vi "Byte_to_DeviceConfigType.vi"(4 "Byte Array":u8[](array[numeric])) -> (1 "output cluster":T1)   [LabVIEW 2020]
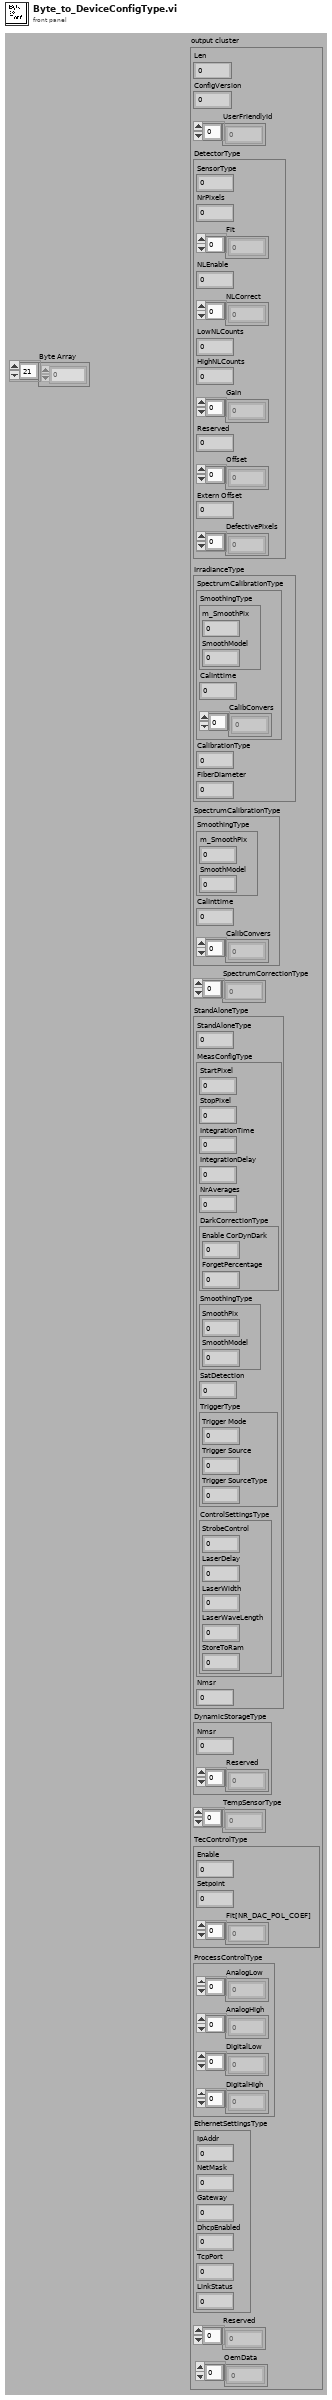
[diagram p1: front panel]
types:
  T1 = cluster{"Len":u16, "ConfigVersion":u16, "UserFriendlyId":u8[], "DetectorType":cluster{"SensorType":u8, "NrPixels":u16, "Fit":sgl[], "NLEnable":u8, "NLCorrect":dbl[], "LowNLCounts":dbl, "HighNLCounts":dbl, "Gain":sgl[], "Reserved":sgl, "Offset":sgl[], "Extern Offset":sgl, "DefectivePixels":u16[]}, "IrradianceType":cluster{"SpectrumCalibrationType":cluster{"SmoothingType":cluster{"m_SmoothPix":u16, "SmoothModel":u8}, "CalInttime":sgl, "CalibConvers":sgl[]}, "CalibrationType":u8, "FiberDiameter":i32}, "SpectrumCalibrationType":cluster{"SmoothingType":cluster{"m_SmoothPix":u16, "SmoothModel":u8}, "CalInttime":sgl, "CalibConvers":sgl[]}, "SpectrumCorrectionType":sgl[], "StandAloneType":cluster{"StandAloneType":u8, "MeasConfigType":cluster{"StartPixel":u16, "StopPixel":u16, "IntegrationTime":sgl, "IntegrationDelay":u32, "NrAverages":u32, "DarkCorrectionType":cluster{"Enable CorDynDark":u8, "ForgetPercentage":u8}, "SmoothingType":cluster{"SmoothPix":u16, "SmoothModel":u8}, "SatDetection":u8, "TriggerType":cluster{"Trigger Mode":u8, "Trigger Source":u8, "Trigger SourceType":u8}, "ControlSettingsType":cluster{"StrobeControl":u16, "LaserDelay":u32, "LaserWidth":u32, "LaserWaveLength":sgl, "StoreToRam":u16}}, "Nmsr":i16}, "DynamicStorageType":cluster{"Nmsr":i32, "Reserved":u8[]}, "TempSensorType":sgl[], "TecControlType":cluster{"Enable":u8, "Setpoint":sgl, "Fit[NR_DAC_POL_COEF]":sgl[]}, "ProcessControlType":cluster{"AnalogLow":sgl[], "AnalogHigh":sgl[], "DigitalLow":sgl[], "DigitalHigh":sgl[]}, "EthernetSettingsType":cluster{"IpAddr":u32, "NetMask":u32, "Gateway":u32, "DhcpEnabled":u8, "TcpPort":u16, "LinkStatus":u8}, "Reserved":u8[], "OemData":u8[]}
  T2 = cluster{"Len":u16, "ConfigVersion":u16, "UserFriendlyId":u8[], "DetectorType":cluster{"SensorType":u8, "NrPixels":u16, "Fit":sgl[], "NLEnable":u8, "NLCorrect":dbl[], "LowNLCounts":dbl, "HighNLCounts":dbl, "Gain":sgl[], "Reserved":sgl, "Offset":sgl[], "Extern Offset":sgl, "DefectivePixels":u16[]}, "IrradianceType":cluster{"SpectrumCalibrationType":cluster{"SmoothingType":cluster{"m_SmoothPix":u16, "SmoothModel":u8}, "CalInttime":sgl, "CalibConvers":sgl[]}, "CalibrationType":u8, "FiberDiameter":i32}, "SpectrumCalibrationType":cluster{"SmoothingType":cluster{"m_SmoothPix":u16, "SmoothModel":u8}, "CalInttime":sgl, "CalibConvers":sgl[]}, "SpectrumCorrectionType":sgl[], "StandAloneType":cluster{"StandAloneType":u8, "MeasConfigType":cluster{"StartPixel":u16, "StopPixel":u16, "IntegrationTime":sgl, "IntegrationDelay":u32, "NrAverages":u32, "DarkCorrectionType":cluster{"Enable CorDynDark":u8, "ForgetPercentage":u8}, "SmoothingType":cluster{"SmoothPix":u16, "SmoothModel":u8}, "SatDetection":u8, "TriggerType":cluster{"Trigger Mode":u8, "Trigger Source":u8, "Trigger SourceType":u8}, "ControlSettingsType":cluster{"StrobeControl":u16, "LaserDelay":u32, "LaserWidth":u32, "LaserWaveLength":sgl, "StoreToRam":u16}}, "Nmsr":i16}, "DynamicStorageType":cluster{"Nmsr":i32, "Reserved":u8[]}, "TempSensorType":sgl[], "TecControlType":cluster{"Enable":u8, "Setpoint":sgl, "Fit[NR_DAC_POL_COEF]":sgl[]}, "ProcessControlType\n":cluster{"AnalogLow":sgl[], "AnalogHigh":sgl[], "DigitalLow":sgl[], "DigitalHigh":sgl[]}, "EthernetSettingsType":cluster{"IpAddr":u32, "NetMask":u32, "Gateway":u32, "DhcpEnabled":u8, "TcpPort":u16, "LinkStatus":u8}, "Reserved":u8[], "OemData":u8[]}
  T3 = cluster{u8, u16, sgl[], u8, dbl[], dbl, dbl, sgl[], sgl, sgl[], sgl, u16[]}
  T4 = cluster{cluster{cluster{u16, u8}, sgl, sgl[]}, u8, i32}
  T5 = cluster{u16, u16, sgl, u32, u32, cluster{u8, u8}, cluster{u16, u8}, u8, cluster{u8, u8, u8}, cluster{u16, u32, u32, sgl, u16}}
  T6 = cluster{u8, cluster{u16, u16, sgl, u32, u32, cluster{u8, u8}, cluster{u16, u8}, u8, cluster{u8, u8, u8}, cluster{u16, u32, u32, sgl, u16}}, i16}
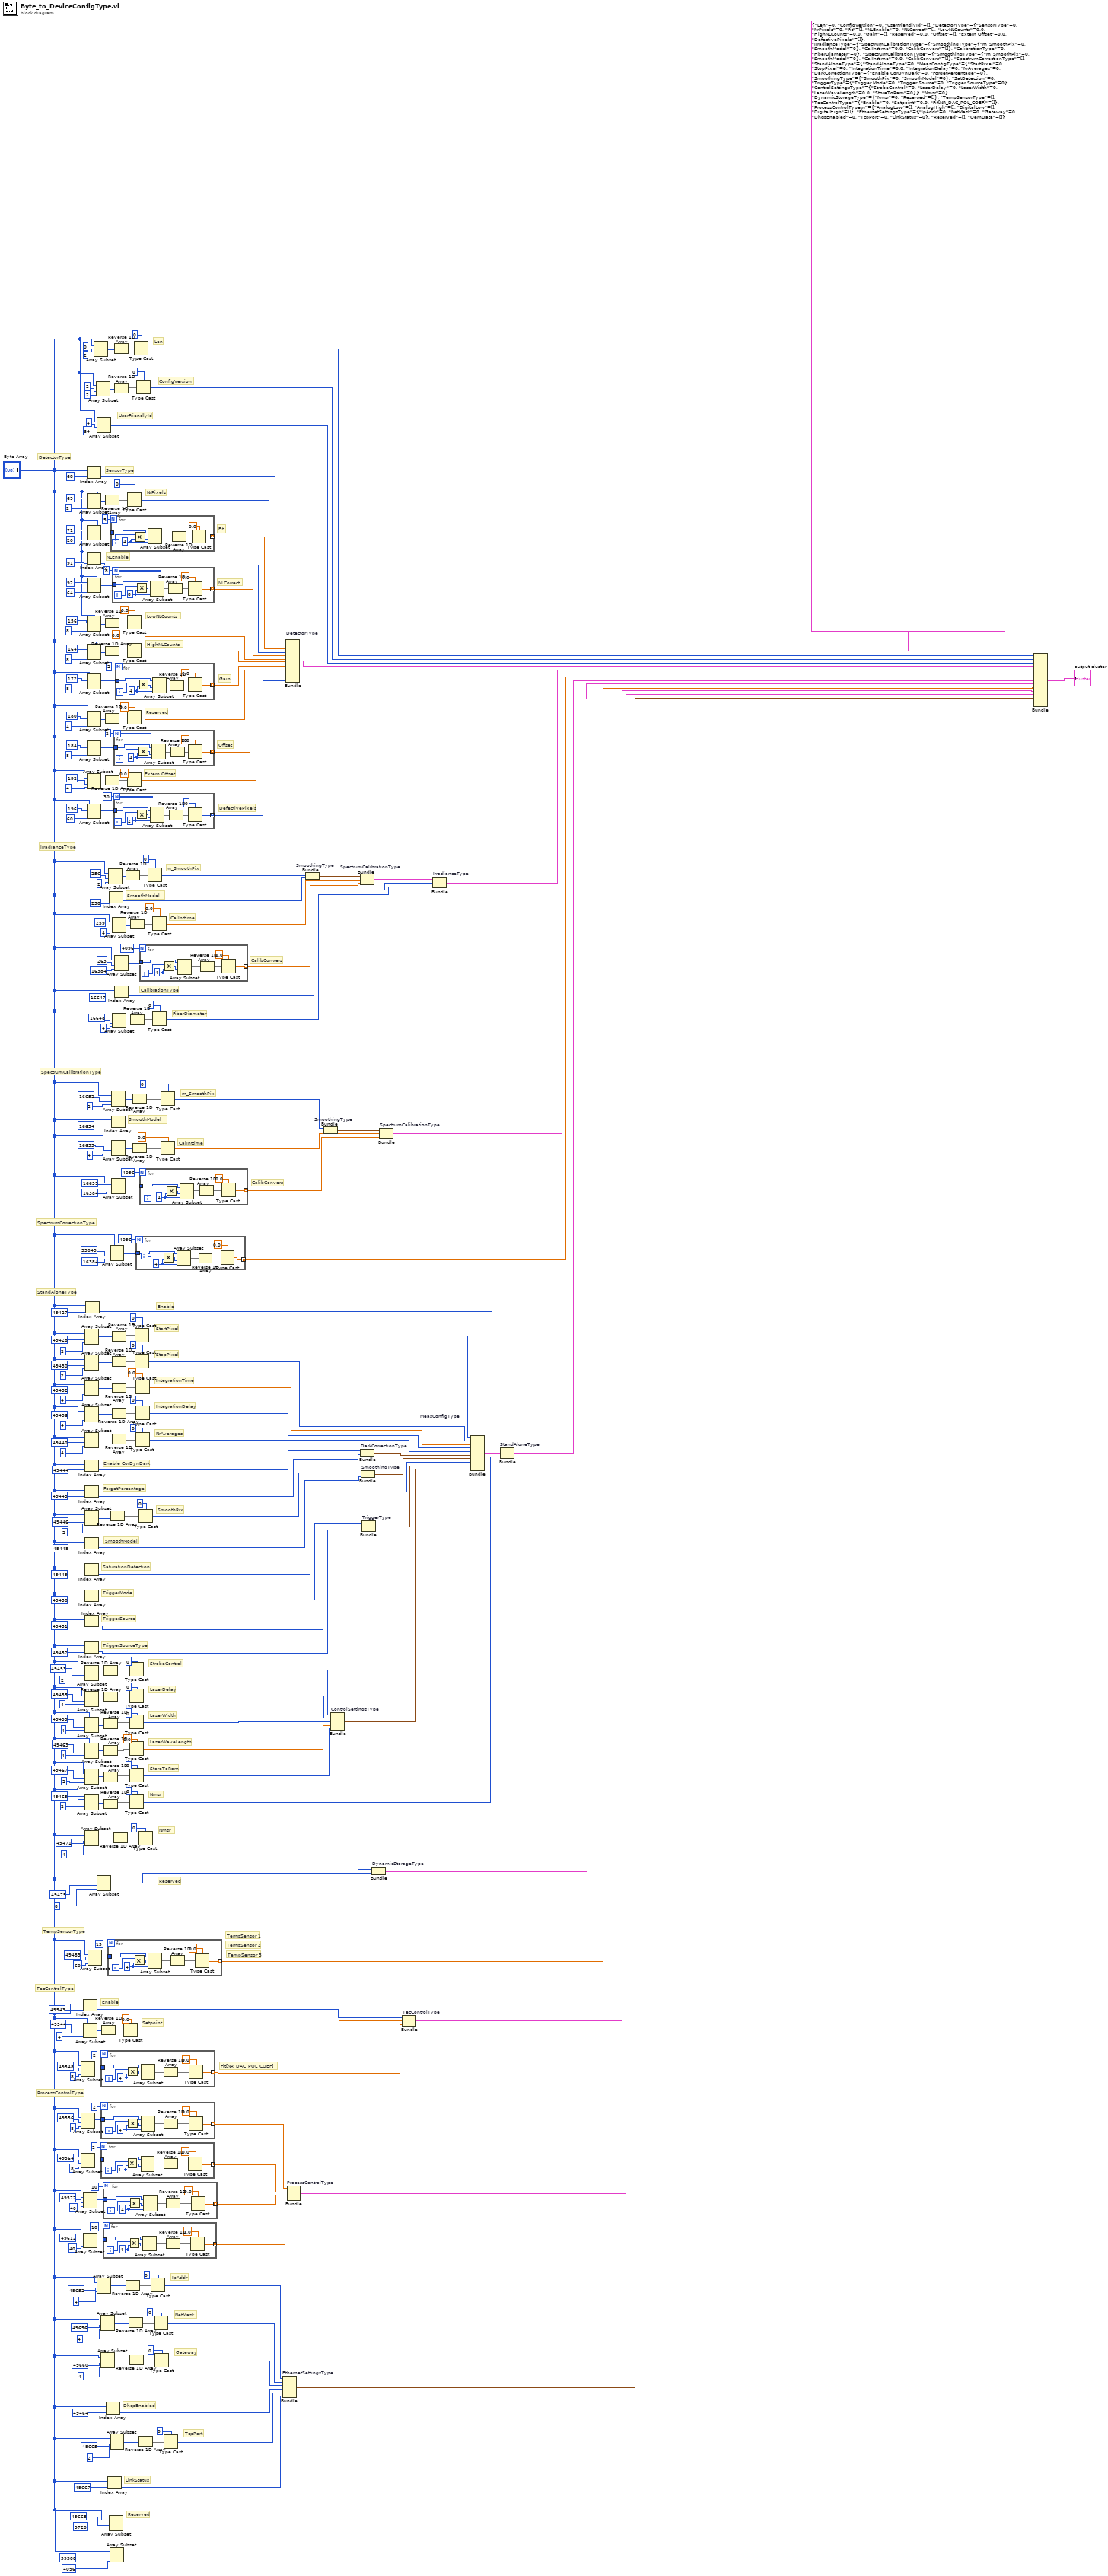
[diagram p0: block diagram]
diagram:
  # "Enable"
  # "LinkStatus"
  # "DhcpEnabled"
  # "TcpPort"
  # "Gateway"
  # "NetMask"
  # "IpAddr"
  # "ProcessControlType"
  # "TecControlType"
  # "Len"
  # "ConfigVersion"
  # "Fit[NR_DAC_POL_COEF]"
  # "Setpoint"
  # "Enable"
  # "UserFriendlyId"
  # "SensorType"
  # "NrPixels"
  # "Fit"
  # "NLEnable"
  # "NLCorrect"
  # "LowNLCounts"
  # "HighNLCounts"
  # "Gain"
  # "Offset"
  # "DetectorType"
  # "TempSensor 3"
  # "TempSensor 2"
  # "Reserved"
  # "TempSensor 1"
  # "TempSensorType"
  # "Reserved"
  # "Nmsr"
  # "Nmsr"
  # "StoreToRam"
  # "LaserWaveLength"
  # "LaserWidth"
  # "LaserDelay"
  # "StrobeControl"
  # "TriggerSourceType"
  # "TriggerSource"
  # "TriggerMode"
  # "SaturationDetection"
  # "SmoothModel"
  # "SmoothPix"
  # "ForgetPercentage"
  # "Enable CorDynDark"
  # "NrAverages"
  # "IntegrationDelay"
  # "IntegrationTime"
  # "StopPixel"
  # "StartPixel"
  # "StandAloneType"
  # "SpectrumCorrectionType"
  # "CalibConvers"
  # "CalInttime"
  # "SmoothModel"
  # "m_SmoothPix"
  # "SpectrumCalibrationType"
  # "FiberDiameter"
  # "CalibrationType"
  # "CalibConvers"
  # "CalInttime"
  # "SmoothModel"
  # "IrradianceType"
  # "m_SmoothPix"
  # "DefectivePixels"
  # "Reserved"
  # "Extern Offset"
  n1 = Array Subset(array="Byte Array", index=49564, length=8) -> (w62:u8[])
  n2 = Array Subset(array="Byte Array", index=49548, length=8) -> (w71:u8[])
  n3 = Array Subset(array="Byte Array", index=49556, length=8) -> (w66:u8[])
  n4 = Index Array(array="Byte Array", index=49543 ("length")) -> (element=w78:u8)
  n5 = Array Subset(array="Byte Array", index=49612, length=40) -> (w54:u8[])
  n6 = Array Subset(array="Byte Array", index=49544, length=4) -> (w74:u8[])
  n7 = Array Subset(array="Byte Array", index=49572, length=40) -> (w58:u8[])
  n8 = Array Subset(array="Byte Array", index=49471 ("length"), length=4) -> (w45:u8[])
  n9 = Array Subset(array="Byte Array", index=49428, length=2) -> (w222:u8[])
  n10 = Array Subset(array="Byte Array", index=49430, length=2) -> (w217:u8[])
  n11 = Array Subset(array="Byte Array", index=49432, length=4) -> (w214:u8[])
  n12 = Array Subset(array="Byte Array", index=49436, length=4) -> (w205:u8[])
  n13 = Array Subset(array="Byte Array", index=49440, length=4) -> (w202:u8[])
  n14 = Index Array(array="Byte Array", index=49444 ("length")) -> (element=w97:u8)
  n15 = Index Array(array="Byte Array", index=49445 ("length")) -> (element=w96:u8)
  n16 = Array Subset(array="Byte Array", index=49446, length=2) -> (w196:u8[])
  n17 = Index Array(array="Byte Array", index=49448 ("length")) -> (element=w94:u8)
  n18 = Index Array(array="Byte Array", index=49449 ("length")) -> (element=w93:u8)
  n19 = Index Array(array="Byte Array", index=49450 ("length")) -> (element=w92:u8)
  n20 = Index Array(array="Byte Array", index=49451 ("length")) -> (element=w91:u8)
  n21 = Index Array(array="Byte Array", index=49452 ("length")) -> (element=w90:u8)
  n22 = Array Subset(array="Byte Array", index=49453, length=2) -> (w184:u8[])
  n23 = Array Subset(array="Byte Array", index=49455, length=4) -> (w181:u8[])
  n24 = Array Subset(array="Byte Array", index=49459, length=4) -> (w174:u8[])
  n25 = Array Subset(array="Byte Array", index=49463, length=4) -> (w171:u8[])
  n26 = Array Subset(array="Byte Array", index=49467, length=2) -> (w164:u8[])
  n27 = Array Subset(array="Byte Array", index=49469, length=2) -> (w159:u8[])
  n28 = Index Array(array="Byte Array", index=49427 ("length")) -> (element=w103:u8)
  n29 = Index Array(array="Byte Array", index=68 ("length")) -> (element=w136:u8)
  n30 = Array Subset(array="Byte Array", index=69, length=2) -> (w300:u8[])
  n31 = Array Subset(array="Byte Array", index=71, length=20) -> (w133:u8[])
  n32 = Index Array(array="Byte Array", index=91 ("length")) -> (element=w132:u8)
  n33 = Array Subset(array="Byte Array", index=92, length=64) -> (w130:u8[])
  n34 = Array Subset(array="Byte Array", index=156, length=8) -> (w286:u8[])
  n35 = Array Subset(array="Byte Array", index=164, length=8) -> (w283:u8[])
  n36 = Array Subset(array="Byte Array", index=172, length=8) -> (w126:u8[])
  n37 = Array Subset(array="Byte Array", index=180, length=4) -> (w274:u8[])
  n38 = Array Subset(array="Byte Array", index=184, length=8) -> (w123:u8[])
  n39 = Array Subset(array="Byte Array", index=192, length=4) -> (w266:u8[])
  n40 = Array Subset(array="Byte Array", index=196, length=60) -> (w121:u8[])
  n41 = Array Subset(array="Byte Array", index=49483, length=60) -> (w81:u8[])
  n42 = Array Subset(array="Byte Array", index=0, length=2) -> (w305:u8[])
  n43 = Array Subset(array="Byte Array", index=2, length=2) -> (w304:u8[])
  n44 = Array Subset(array="Byte Array", index=4, length=64) -> (w137:u8[])
  n45 = Array Subset(array="Byte Array", index=49475, length=8) -> (w80:u8[])
  n46 = Array Subset(array="Byte Array", index=49652 ("length"), length=4) -> (w38:u8[])
  n47 = for {
    N: 2 -> [_]
    tunnel: w62 -> [w318]
    tunnel: [w316] -> w49 mode=indexing
    i -> [w319]
    w320 = 4 ("length")
    n48 = Multiply(x=w319, y=w320) -> (x*y=w321:i32)
    n49 = Array Subset(array=w318, index=w321, length=w320) -> (w314:u8[])
    n50 = Reverse 1D Array(array=w314) -> (reversed array=w315:u8[])
    n51 = Type Cast(type=sgl 0.0, x=w315) -> (*(type *) &x=w316:sgl)
  }
  n52 = Array Subset(array="Byte Array", index=49656 ("length"), length=4) -> (w33:u8[])
  n53 = for {
    N: 2 -> [_]
    tunnel: w71 -> [w326]
    tunnel: [w324] -> w67 mode=indexing
    i -> [w327]
    w328 = 4 ("length")
    n54 = Multiply(x=w327, y=w328) -> (x*y=w329:i32)
    n55 = Array Subset(array=w326, index=w329, length=w328) -> (w322:u8[])
    n56 = Reverse 1D Array(array=w322) -> (reversed array=w323:u8[])
    n57 = Type Cast(type=sgl 0.0, x=w323) -> (*(type *) &x=w324:sgl)
  }
  n58 = for {
    N: 2 -> [_]
    tunnel: w66 -> [w334]
    tunnel: [w332] -> w50 mode=indexing
    i -> [w335]
    w336 = 4 ("length")
    n59 = Multiply(x=w335, y=w336) -> (x*y=w337:i32)
    n60 = Array Subset(array=w334, index=w337, length=w336) -> (w330:u8[])
    n61 = Reverse 1D Array(array=w330) -> (reversed array=w331:u8[])
    n62 = Type Cast(type=sgl 0.0, x=w331) -> (*(type *) &x=w332:sgl)
  }
  n63 = Array Subset(array="Byte Array", index=49660 ("length"), length=4) -> (w28:u8[])
  n64 = Reverse 1D Array(array=w74) -> (reversed array=w73:u8[])
  n65 = for {
    N: 10 -> [_]
    tunnel: w54 -> [w342]
    tunnel: [w340] -> w47 mode=indexing
    i -> [w343]
    w344 = 4 ("length")
    n66 = Multiply(x=w343, y=w344) -> (x*y=w345:i32)
    n67 = Array Subset(array=w342, index=w345, length=w344) -> (w338:u8[])
    n68 = Reverse 1D Array(array=w338) -> (reversed array=w339:u8[])
    n69 = Type Cast(type=sgl 0.0, x=w339) -> (*(type *) &x=w340:sgl)
  }
  n70 = for {
    N: 10 -> [_]
    tunnel: w58 -> [w350]
    tunnel: [w348] -> w48 mode=indexing
    i -> [w351]
    w352 = 4 ("length")
    n71 = Multiply(x=w351, y=w352) -> (x*y=w353:i32)
    n72 = Array Subset(array=w350, index=w353, length=w352) -> (w346:u8[])
    n73 = Reverse 1D Array(array=w346) -> (reversed array=w347:u8[])
    n74 = Type Cast(type=sgl 0.0, x=w347) -> (*(type *) &x=w348:sgl)
  }
  n75 = Reverse 1D Array(array=w184) -> (reversed array=w183:u8[])
  n76 = Reverse 1D Array(array=w181) -> (reversed array=w182:u8[])
  n77 = Reverse 1D Array(array=w174) -> (reversed array=w173:u8[])
  n78 = Reverse 1D Array(array=w171) -> (reversed array=w172:u8[])
  n79 = Reverse 1D Array(array=w164) -> (reversed array=w165:u8[])
  n80 = Reverse 1D Array(array=w159) -> (reversed array=w158:u8[])
  n81 = Reverse 1D Array(array=w300) -> (reversed array=w301:u8[])
  n82 = Reverse 1D Array(array=w286) -> (reversed array=w285:u8[])
  n83 = Reverse 1D Array(array=w283) -> (reversed array=w284:u8[])
  n84 = Reverse 1D Array(array=w274) -> (reversed array=w273:u8[])
  n85 = Reverse 1D Array(array=w266) -> (reversed array=w267:u8[])
  n86 = Index Array(array="Byte Array", index=49464 ("length")) -> (element=w14:u8)
  n87 = for {
    N: 15 -> [_]
    tunnel: w81 -> [w358]
    tunnel: [w356] -> w7 mode=indexing
    i -> [w359]
    w360 = 4 ("length")
    n88 = Multiply(x=w359, y=w360) -> (x*y=w361:i32)
    n89 = Array Subset(array=w358, index=w361, length=w360) -> (w354:u8[])
    n90 = Reverse 1D Array(array=w354) -> (reversed array=w355:u8[])
    n91 = Type Cast(type=sgl 0.0, x=w355) -> (*(type *) &x=w356:sgl)
  }
  n92 = Index Array(array="Byte Array", index=49667 ("length")) -> (element=w12:u8)
  n93 = Array Subset(array="Byte Array", index=256, length=2) -> (w257:u8[])
  n94 = Index Array(array="Byte Array", index=258 ("length")) -> (element=w118:u8)
  n95 = Array Subset(array="Byte Array", index=49668, length=9720) -> (w11:u8[])
  n96 = Array Subset(array="Byte Array", index=59388, length=4096) -> (w3:u8[])
  n97 = for {
    N: 5 -> [_]
    tunnel: w133 -> [w366]
    tunnel: [w364] -> w134 mode=indexing
    i -> [w367]
    w368 = 4 ("length")
    n98 = Multiply(x=w367, y=w368) -> (x*y=w369:i32)
    n99 = Array Subset(array=w366, index=w369, length=w368) -> (w363:u8[])
    n100 = Reverse 1D Array(array=w363) -> (reversed array=w362:u8[])
    n101 = Type Cast(type=sgl 0.0, x=w362) -> (*(type *) &x=w364:sgl)
  }
  n102 = Array Subset(array="Byte Array", index=33043, length=16384) -> (w89:u8[])
  n103 = Array Subset "Array Subset"(array="Byte Array", index=49665 ("length"), length=2) -> (w20:u8[])
  n104 = Reverse 1D Array(array=w196) -> (reversed array=w197:u8[])
  n105 = Array Subset(array="Byte Array", index=16652, length=2) -> (w231:u8[])
  n106 = Index Array(array="Byte Array", index=16654 ("length")) -> (element=w110:u8)
  n107 = Array Subset(array="Byte Array", index=16655, length=4) -> (w234:u8[])
  n108 = Array Subset(array="Byte Array", index=16659, length=16384) -> (w88:u8[])
  n109 = Reverse 1D Array(array=w222) -> (reversed array=w223:u8[])
  n110 = Reverse 1D Array(array=w217) -> (reversed array=w216:u8[])
  n111 = Reverse 1D Array(array=w214) -> (reversed array=w215:u8[])
  n112 = Reverse 1D Array(array=w205) -> (reversed array=w204:u8[])
  n113 = Reverse 1D Array(array=w202) -> (reversed array=w203:u8[])
  n114 = for {
    N: 8 -> [_]
    tunnel: w130 -> [w374]
    tunnel: [w372] -> w131 mode=indexing
    i -> [w375]
    w376 = 8 ("length")
    n115 = Multiply(x=w375, y=w376) -> (x*y=w377:i32)
    n116 = Array Subset(array=w374, index=w377, length=w376) -> (w371:u8[])
    n117 = Reverse 1D Array(array=w371) -> (reversed array=w370:u8[])
    n118 = Type Cast(type=0.0, x=w370) -> (*(type *) &x=w372:dbl)
  }
  n119 = Array Subset(array="Byte Array", index=259, length=4) -> (w253:u8[])
  n120 = Array Subset(array="Byte Array", index=16648, length=4) -> (w244:u8[])
  n121 = for {
    N: 30 -> [_]
    tunnel: w121 -> [w382]
    tunnel: [w380] -> w120 mode=indexing
    i -> [w383]
    w384 = 2 ("length")
    n122 = Multiply(x=w383, y=w384) -> (x*y=w385:i32)
    n123 = Array Subset(array=w382, index=w385, length=w384) -> (w379:u8[])
    n124 = Reverse 1D Array(array=w379) -> (reversed array=w378:u8[])
    n125 = Type Cast(type=u16 0, x=w378) -> (*(type *) &x=w380:u16)
  }
  n126 = Reverse 1D Array(array=w45) -> (reversed array=w46:u8[])
  n127 = for {
    N: 2 -> [_]
    tunnel: w123 -> [w390]
    tunnel: [w388] -> w124 mode=indexing
    i -> [w391]
    w392 = 4 ("length")
    n128 = Multiply(x=w391, y=w392) -> (x*y=w393:i32)
    n129 = Array Subset(array=w390, index=w393, length=w392) -> (w387:u8[])
    n130 = Reverse 1D Array(array=w387) -> (reversed array=w386:u8[])
    n131 = Type Cast(type=sgl 0.0, x=w386) -> (*(type *) &x=w388:sgl)
  }
  n132 = Array Subset(array="Byte Array", index=263, length=16384) -> (w116:u8[])
  n133 = Reverse 1D Array(array=w305) -> (reversed array=w148:u8[])
  n134 = Reverse 1D Array(array=w304) -> (reversed array=w303:u8[])
  n135 = Index Array(array="Byte Array", index=16647 ("length")) -> (element=w114:u8)
  n136 = for {
    N: 2 -> [_]
    tunnel: w126 -> [w398]
    tunnel: [w396] -> w127 mode=indexing
    i -> [w399]
    w400 = 4 ("length")
    n137 = Multiply(x=w399, y=w400) -> (x*y=w401:i32)
    n138 = Array Subset(array=w398, index=w401, length=w400) -> (w395:u8[])
    n139 = Reverse 1D Array(array=w395) -> (reversed array=w394:u8[])
    n140 = Type Cast(type=sgl 0.0, x=w394) -> (*(type *) &x=w396:sgl)
  }
  n141 = Type Cast(type=sgl 0.0, x=w73) -> (*(type *) &x=w72:sgl)
  n142 = Reverse 1D Array(array=w38) -> (reversed array=w39:u8[])
  n143 = Reverse 1D Array(array=w257) -> (reversed array=w256:u8[])
  n144 = Type Cast(type=u16 0, x=w301) -> (*(type *) &x=w135:u16)
  n145 = Type Cast(type=0.0, x=w285) -> (*(type *) &x=w129:dbl)
  n146 = Type Cast(type=0.0, x=w284) -> (*(type *) &x=w128:dbl)
  n147 = Type Cast(type=sgl 0.0, x=w273) -> (*(type *) &x=w125:sgl)
  n148 = Type Cast(type=sgl 0.0, x=w267) -> (*(type *) &x=w122:sgl)
  n149 = Reverse 1D Array(array=w33) -> (reversed array=w34:u8[])
  n150 = Type Cast(type=u16 0, x=w183) -> (*(type *) &x=w87:u16)
  n151 = Type Cast(type=u32 0, x=w182) -> (*(type *) &x=w86:u32)
  n152 = Type Cast(type=u32 0, x=w173) -> (*(type *) &x=w85:u32)
  n153 = Type Cast(type=sgl 0.0, x=w172) -> (*(type *) &x=w84:sgl)
  n154 = Type Cast(type=u16 0, x=w165) -> (*(type *) &x=w83:u16)
  n155 = Type Cast(type=i16 0, x=w158) -> (*(type *) &x=w82:i16)
  n156 = Reverse 1D Array(array=w28) -> (reversed array=w29:u8[])
  n157 = Reverse 1D Array(array=w253) -> (reversed array=w254:u8[])
  n158 = Reverse 1D Array(array=w244) -> (reversed array=w245:u8[])
  n159 = Reverse 1D Array(array=w231) -> (reversed array=w149:u8[])
  n160 = Reverse 1D Array(array=w234) -> (reversed array=w233:u8[])
  n161 = Type Cast(type=u16 0, x=w148) -> (*(type *) &x=w139:u16)
  n162 = Type Cast(type=u16 0, x=w223) -> (*(type *) &x=w102:u16)
  n163 = Type Cast(type=u16 0, x=w216) -> (*(type *) &x=w101:u16)
  n164 = Type Cast(type=sgl 0.0, x=w215) -> (*(type *) &x=w100:sgl)
  n165 = Type Cast(type=u32 0, x=w204) -> (*(type *) &x=w99:u32)
  n166 = Type Cast(type=u32 0, x=w203) -> (*(type *) &x=w98:u32)
  n167 = for {
    N: 4096 -> [_]
    tunnel: w89 -> [w406]
    tunnel: [w404] -> w105 mode=indexing
    i -> [w407]
    w408 = 4 ("length")
    n168 = Multiply(x=w407, y=w408) -> (x*y=w409:i32)
    n169 = Array Subset(array=w406, index=w409, length=w408) -> (w403:u8[])
    n170 = Reverse 1D Array(array=w403) -> (reversed array=w402:u8[])
    n171 = Type Cast(type=sgl 0.0, x=w402) -> (*(type *) &x=w404:sgl)
  }
  n172 = Type Cast(type=u16 0, x=w303) -> (*(type *) &x=w138:u16)
  n173 = Type Cast(type=u32 0, x=w46) -> (*(type *) &x=w42:u32)
  n174 = Type Cast(type=u16 0, x=w197) -> (*(type *) &x=w95:u16)
  n175 = Reverse 1D Array(array=w20) -> (reversed array=w21:u8[])
  n176 = for {
    N: 4096 -> [_]
    tunnel: w116 -> [w414]
    tunnel: [w412] -> w115 mode=indexing
    i -> [w415]
    w416 = 4 ("length")
    n177 = Multiply(x=w415, y=w416) -> (x*y=w417:i32)
    n178 = Array Subset(array=w414, index=w417, length=w416) -> (w411:u8[])
    n179 = Reverse 1D Array(array=w411) -> (reversed array=w410:u8[])
    n180 = Type Cast(type=sgl 0.0, x=w410) -> (*(type *) &x=w412:sgl)
  }
  n181 = for {
    N: 4096 -> [_]
    tunnel: w88 -> [w422]
    tunnel: [w420] -> w108 mode=indexing
    i -> [w423]
    w424 = 4 ("length")
    n182 = Multiply(x=w423, y=w424) -> (x*y=w425:i32)
    n183 = Array Subset(array=w422, index=w425, length=w424) -> (w419:u8[])
    n184 = Reverse 1D Array(array=w419) -> (reversed array=w418:u8[])
    n185 = Type Cast(type=sgl 0.0, x=w418) -> (*(type *) &x=w420:sgl)
  }
  n186 = Type Cast(type=u16 0, x=w256) -> (*(type *) &x=w119:u16)
  n187 = Type Cast(type=u32 0, x=w39) -> (*(type *) &x=w24:u32)
  n188 = Type Cast(type=sgl 0.0, x=w254) -> (*(type *) &x=w117:sgl)
  n189 = Type Cast(type=0, x=w245) -> (*(type *) &x=w113:i32)
  n190 = Type Cast(type=u32 0, x=w34) -> (*(type *) &x=w23:u32)
  n191 = Type Cast(type=u32 0, x=w29) -> (*(type *) &x=w22:u32)
  n192 = Type Cast(type=u16 0, x=w149) -> (*(type *) &x=w111:u16)
  n193 = Type Cast(type=sgl 0.0, x=w233) -> (*(type *) &x=w109:sgl)
  n194 = Type Cast(type=u16 0, x=w21) -> (*(type *) &x=w13:u16)
  n195 = Bundle "EthernetSettingsType"(w24, w23, w22, w14, w13, w12) -> (w10:cluster{u32, u32, u32, u8, u16, u8})  [unwired: 1 in]
  n196 = Bundle "DetectorType"(w136, w135, w134, w132, w131, w129, w128, w127, w125, w124, w122, w120) -> (w147:T3)  [unwired: 1 in]
  n197 = Bundle "ProcessControlType"(w50, w49, w48, w47) -> (w9:cluster{sgl[], sgl[], sgl[], sgl[]})  [unwired: 1 in]
  n198 = Bundle "SmoothingType"(w119, w118) -> (w142:cluster{u16, u8})  [unwired: 1 in]
  n199 = Bundle "SmoothingType"(w111, w110) -> (w112:cluster{u16, u8})  [unwired: 1 in]
  n200 = Bundle "ControlSettingsType"(w87, w86, w85, w84, w83) -> (w140:cluster{u16, u32, u32, sgl, u16})  [unwired: 1 in]
  n201 = Bundle "SpectrumCalibrationType"(w142, w117, w115) -> (w107:cluster{cluster{u16, u8}, sgl, sgl[]})  [unwired: 1 in]
  n202 = Bundle "DarkCorrectionType"(w97, w96) -> (w143:cluster{u8, u8})  [unwired: 1 in]
  n203 = Bundle "SmoothingType"(w95, w94) -> (w104:cluster{u16, u8})  [unwired: 1 in]
  n204 = Bundle "TriggerType"(w92, w91, w90) -> (w141:cluster{u8, u8, u8})  [unwired: 1 in]
  n205 = Bundle "DynamicStorageType"(w42, w80) -> (w6:cluster{u32, u8[]})  [unwired: 1 in]
  n206 = Bundle "SpectrumCalibrationType"(w112, w109, w108) -> (w106:cluster{cluster{u16, u8}, sgl, sgl[]})  [unwired: 1 in]
  n207 = Bundle "TecControlType"(w78, w72, w67) -> (w8:cluster{u8, sgl, sgl[]})  [unwired: 1 in]
  n208 = Bundle "IrradianceType"(w107, w114, w113) -> (w146:T4)  [unwired: 1 in]
  n209 = Bundle "MeasConfigType"(w102, w101, w100, w99, w98, w143, w104, w93, w141, w140) -> (w144:T5)  [unwired: 1 in]
  n210 = Bundle "StandAloneType"(w103, w144, w82) -> (w145:T6)  [unwired: 1 in]
  n211 = Bundle(cluster=T2 {"Len"=0, "ConfigVersion"=0, "UserFriendlyId"=[], "DetectorType"={"SensorType"=0, "NrPixels"=0, "Fit"=[], "NLEnable"=0, "NLCorrect"=[], "LowNLCounts"=0.0, "HighNLCounts"=0.0, "Gain"=[], "Reserved"=0.0, "Offset"=[], "Extern Offset"=0.0, "DefectivePixels"=[]}, "IrradianceType"={"SpectrumCalibrationType"={"SmoothingType"={"m_SmoothPix"=0, "SmoothModel"=0}, "CalInttime"=0.0, "CalibConvers"=[]}, "CalibrationType"=0, "FiberDiameter"=0}, "SpectrumCalibrationType"={"SmoothingType"={"m_SmoothPix"=0, "SmoothModel"=0}, "CalInttime"=0.0, "CalibConvers"=[]}, "SpectrumCorrectionType"=[], "StandAloneType"={"StandAloneType"=0, "MeasConfigType"={"StartPixel"=0, "StopPixel"=0, "IntegrationTime"=0.0, "IntegrationDelay"=0, "NrAverages"=0, "DarkCorrectionType"={"Enable CorDynDark"=0, "ForgetPercentage"=0}, "SmoothingType"={"SmoothPix"=0, "SmoothModel"=0}, "SatDetection"=0, "TriggerType"={"Trigger Mode"=0, "Trigger Source"=0, "Trigger SourceType"=0}, "ControlSettingsType"={"StrobeControl"=0, "LaserDelay"=0, "LaserWidth"=0, "LaserWaveLength"=0.0, "StoreToRam"=0}}, "Nmsr"=0}, "DynamicStorageType"={"Nmsr"=0, "Reserved"=[]}, "TempSensorType"=[], "TecControlType"={"Enable"=0, "Setpoint"=0.0, "Fit[NR_DAC_POL_COEF]"=[]}, "ProcessControlType\n"={"AnalogLow"=[], "AnalogHigh"=[], "DigitalLow"=[], "DigitalHigh"=[]}, "EthernetSettingsType"={"IpAddr"=0, "NetMask"=0, "Gateway"=0, "DhcpEnabled"=0, "TcpPort"=0, "LinkStatus"=0}, "Reserved"=[], "OemData"=[]} ("DeviceConfig"), "Len"=w139, "ConfigVersion"=w138, "UserFriendlyId"=w137, "DetectorType"=w147, "IrradianceType"=w146, "SpectrumCalibrationType"=w106, "SpectrumCorrectionType"=w105, "StandAloneType"=w145, "DynamicStorageType"=w6, "TempSensorType"=w7, "TecControlType"=w8, "ProcessControlType"=w9, "EthernetSettingsType"=w10, "Reserved"=w11, "OemData"=w3) -> (→"output cluster":T2)
